vi "Test DMM Module API.vi"() -> ()   [LabVIEW 2018]
doc: "DMM Module API Tester."
uses:
  DMM Module.lvlib
  Application/Application.lvlib
panel:
  out "range?":string
  in  "query range":bool
  out "func?":string
  in  "Query func":bool
  in  "DMM reset":bool
  in  "DMM connect and reset":bool
  in  "Sets to Display":u16(ring)=2 items=["1st Display", "2nd Display", "1st & 2nd Display"]
  out "DCI":dbl
  out "DCV":dbl
  in  "DMM Close":bool
  in  "Detector Rate":u8(ring)=2 items=["SLOW", "MID", "FAST"]
  in  "DCI range":dbl=0.5 format="%#_13g"
  in  "DCV range":dbl=1000.0
  in  "Read DCV_DCI":bool
  in  "config channel":bool
  in  "DMM name":refnum<visa-resource-name>="COM15"
  in  "Show Block Diagram":bool
  in  "Stop Module":bool
  in  "Start Module":bool
  in  "Hide Module Panel":bool
  in  "Show Module Panel":bool
  out "Status":string
  out "Module Running?":bool
  # "This VI tests the API for the Module."
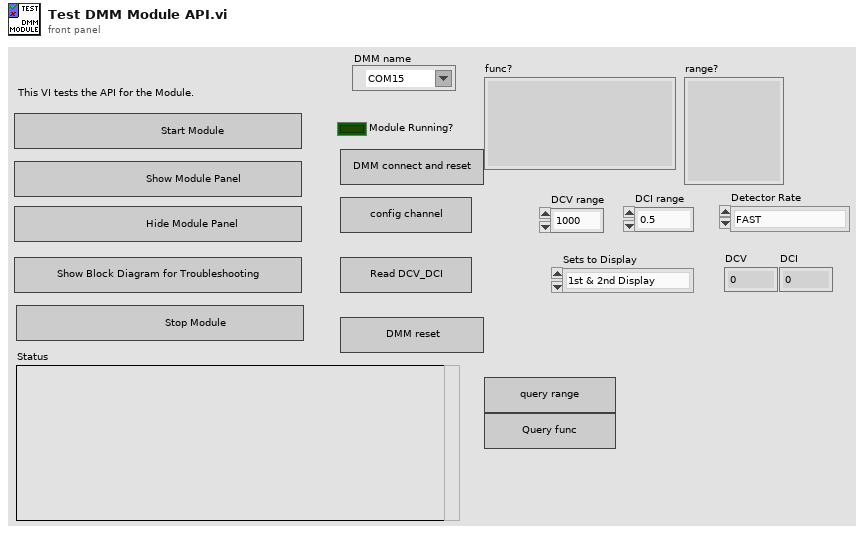
[diagram p1: front panel]
types:
  T1 = typedef "DMM Module.lvlib/Broadcast Events--cluster.ctl" = cluster{"Module Did Init":refnum<user-event>, "Status Updated":refnum<user-event>, "Error Reported":refnum<user-event>, "Module Did Stop":refnum<user-event>, "Update Module Execution Status":refnum<user-event>}
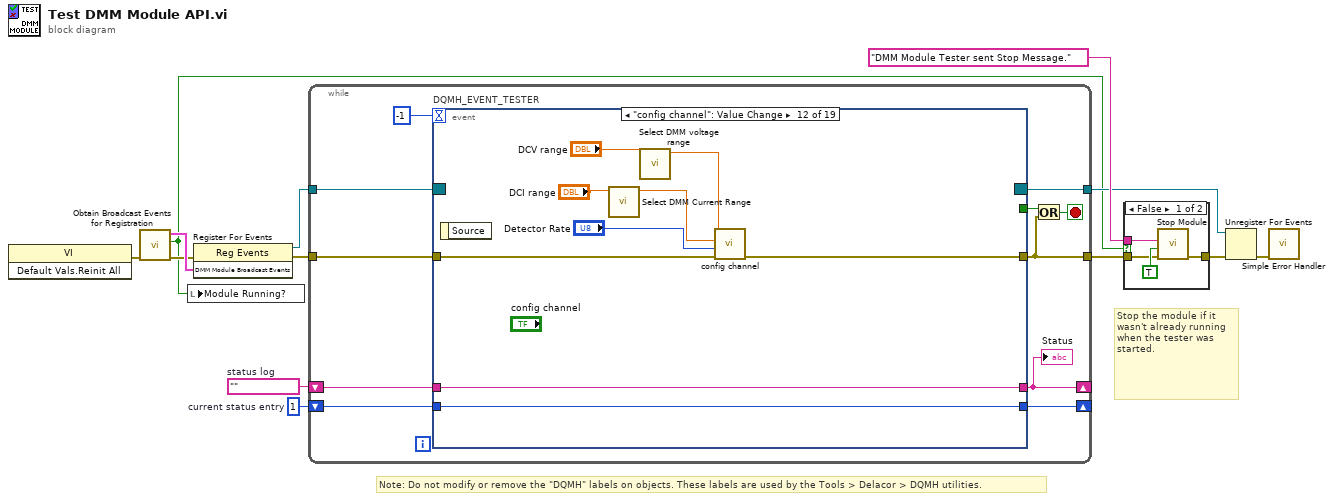
[diagram p0: block diagram]
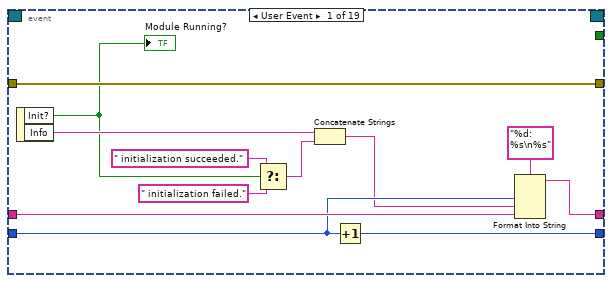
[diagram p3: hidden frame]
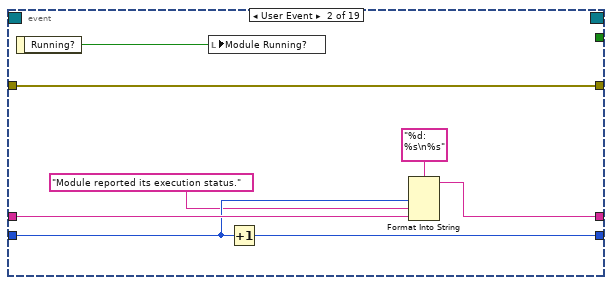
[diagram p4: hidden frame]
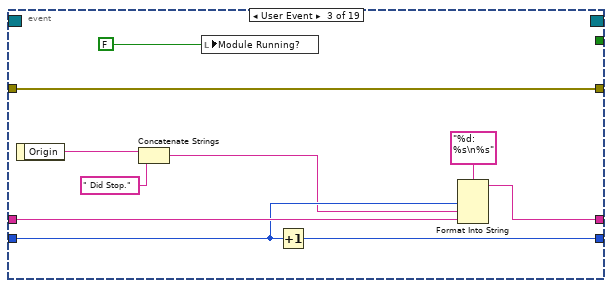
[diagram p5: hidden frame]
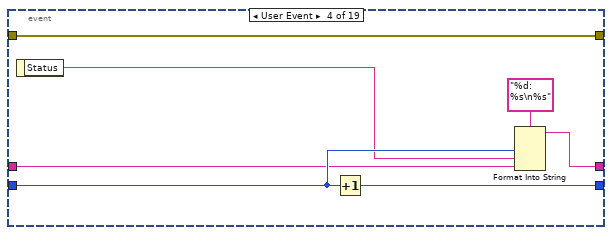
[diagram p6: hidden frame]
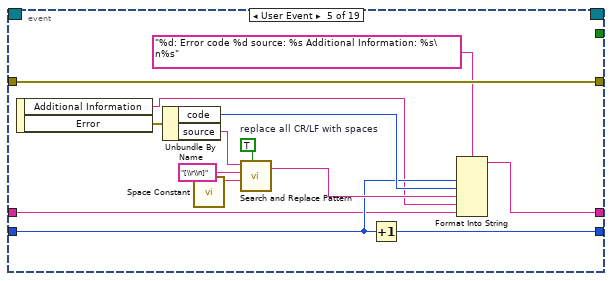
[diagram p7: hidden frame]
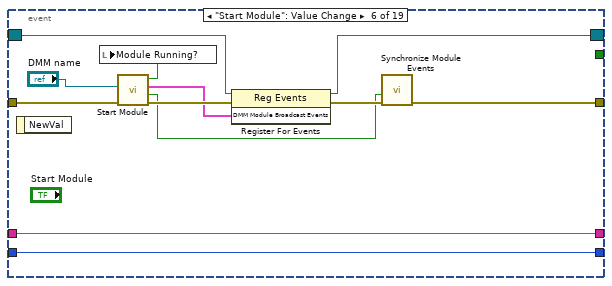
[diagram p8: hidden frame]
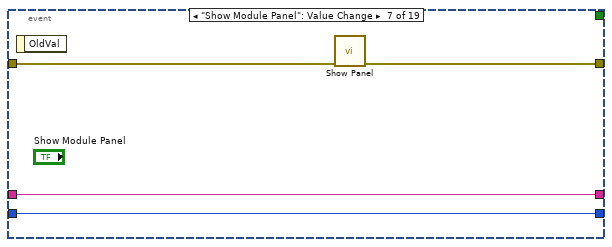
[diagram p9: hidden frame]
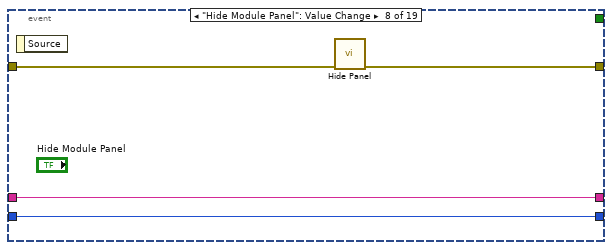
[diagram p10: hidden frame]
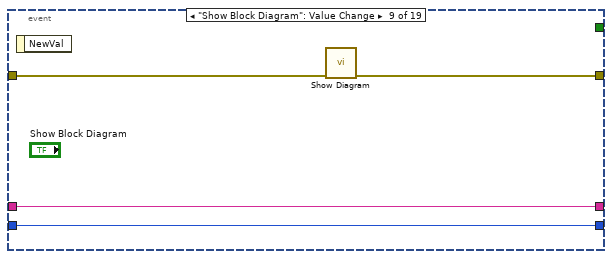
[diagram p11: hidden frame]
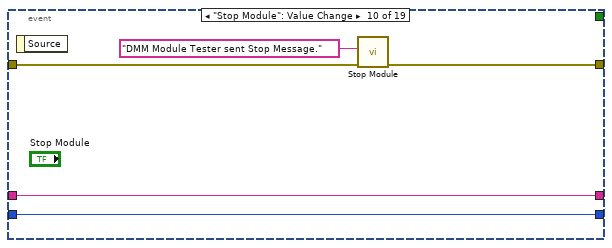
[diagram p12: hidden frame]
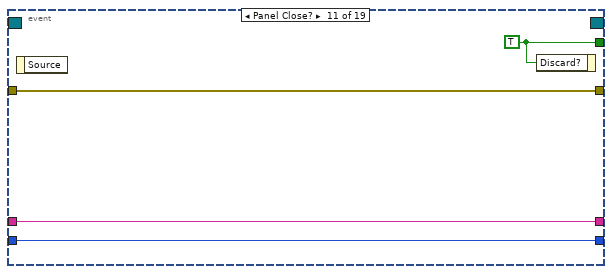
[diagram p13: hidden frame]
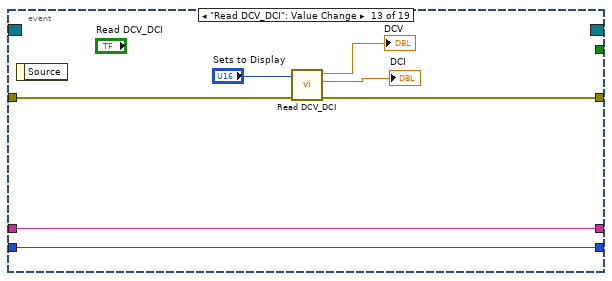
[diagram p14: hidden frame]
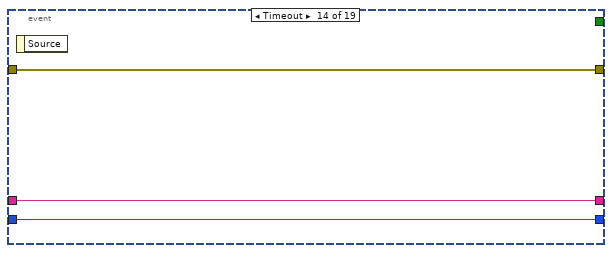
[diagram p15: hidden frame]
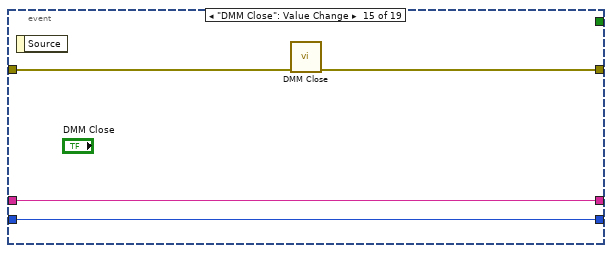
[diagram p16: hidden frame]
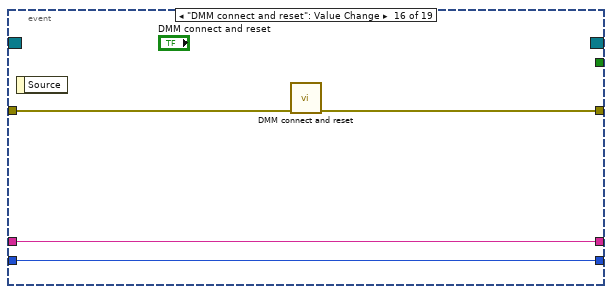
[diagram p17: hidden frame]
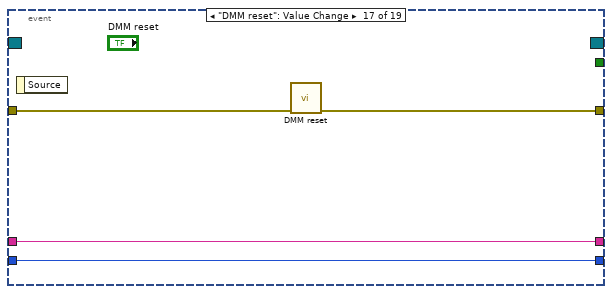
[diagram p18: hidden frame]
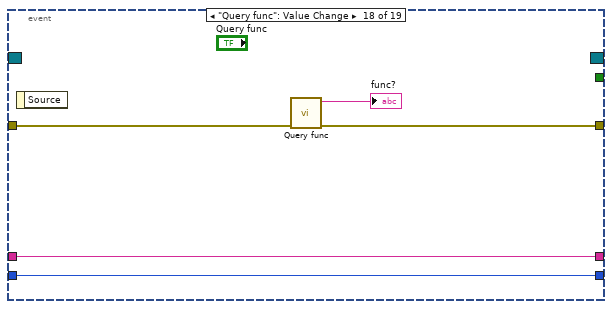
[diagram p19: hidden frame]
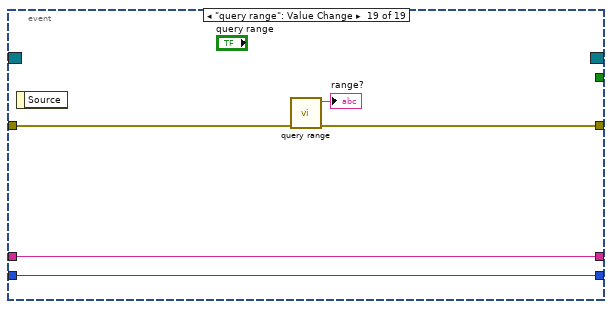
[diagram p20: hidden frame]
diagram:
  w10 = 1  # current status entry
  w11 = ""  # status log
  # "Stop the module if it wasn't already running when the tester was started."
  # "Note: Do not modify or remove the \"DQMH\" labels on objects. These labels are used by the Tools > Delacor > DQMH utilities."
  n1 = invoke class="VI" method="Default Vals.Reinit All"() -> (error out=w5:errorcluster)  [unwired: 3 in, 2 out]
  n2 = call "Obtain Broadcast Events for Registration.vi"("error in (no error)"=w5) -> ("error out"=w4:errorcluster, "Already running?"=w3:bool, "DMM Module Broadcast Events"=w8:T1)  [unwired: 8 in]
  n3 = local write "Module Running?"(w3) -> ()
  n4 = register-events(error in=w4, w8) -> (reference out=w7:refnum<event-registration>, error out=w9:errorcluster)  [unwired: 1 in]
  n5 = while {
    tunnel: w7 -> [w24]
    tunnel: [w15] -> w2
    shift-right: [w19] -> _
    shift-left: w11 -> [w21]
    shift-right: [w20] -> _
    shift-left: w10 -> [w22]
    tunnel: w9 -> [w17]
    tunnel: [w16] -> w6
    stop <- w18 stop-if-true
    n6 = event "DQMH_EVENT_TESTER" shown="[11] \"config channel\": Value Change" {
      selector: w24 -> [_ _ _ _ _ w81 _ _ _ _ _ _ _ _ _ _ _ _ _]
      dyn-events: [_ _ _ _ _ w80 _ _ _ _ _ _ _ _ _ _ _ _ _] -> w16
      timeout: -1 -> [_ _ _ _ _ _ _ _ _ _ _ _ _ _ _ _ _ _ _]
      tunnel: [_ _ _ _ _ _ _ _ _ _ w108 _ _ _ _ _ _ _ _] -> w23
      tunnel: [w36 w38 w45 w55 w75 w79 w91 w95 w96 w102 w105 w114 w118 w125 w128 w132 w136 w141 w146] -> w15
      tunnel: w22 -> [w33 w42 w52 w58 w65 w84 w89 w93 w97 w103 w106 w115 w123 w126 w129 w133 w137 w142 w147]
      tunnel: w21 -> [w34 w43 w53 w57 w63 w85 w90 w94 w98 w104 w107 w116 w124 w127 w130 w134 w138 w143 w148]
      tunnel: [w31 w40 w50 w59 w66 w85 w90 w94 w98 w104 w107 w116 w124 w127 w130 w134 w138 w143 w148] -> w19
      tunnel: [w32 w41 w51 w61 w64 w84 w89 w93 w97 w103 w106 w115 w123 w126 w129 w133 w137 w142 w147] -> w20
      tunnel: w17 -> [w36 w38 w45 w55 w75 w78 w88 w92 w99 w100 w105 w117 w119 w125 w131 w135 w139 w144 w149]
      event User Event {
        n7 = event-data() -> ("Init?"=w28:bool, "Info"=w30:string)  [unwired: 1 in]
        "Module Running?" <- w28
        n8 = Select(t=" initialization succeeded.", s=w28, f=" initialization failed.") -> (s? t:f=w25:string)
        n9 = Concatenate Strings(w30, w25) -> (w29:string)
        n10 = Increment(x=w33) -> (x+1=w32:i32)
        n11 = Format Into String(format string="%d: %s\n%s", w33, w29, w34) -> (resulting string=w31:string)  [unwired: 2 in, 1 out]
      }
      event User Event {
        n12 = event-data() -> ("Running?"=w37:bool)  [unwired: 1 in]
        n13 = local write "Module Running?"(w37) -> ()
        n14 = Increment(x=w42) -> (x+1=w41:i32)
        n15 = Format Into String(format string="%d: %s\n%s", w42, "Module reported its execution status.", w43) -> (resulting string=w40:string)  [unwired: 2 in, 1 out]
      }
      event User Event {
        n16 = event-data() -> ("Origin"=w49:string)  [unwired: 1 in]
        n17 = Concatenate Strings(w49, " Did Stop.") -> (w48:string)
        n18 = local write "Module Running?"(FALSE ("Module Did Init?")) -> ()
        n19 = Increment(x=w52) -> (x+1=w51:i32)
        n20 = Format Into String(format string="%d: %s\n%s", w52, w48, w53) -> (resulting string=w50:string)  [unwired: 2 in, 1 out]
      }
      event User Event {
        n21 = event-data() -> ("Status"=w56:string)  [unwired: 1 in]
        n22 = Increment(x=w58) -> (x+1=w61:i32)
        n23 = Format Into String(format string="%d: %s\n%s", w58, w56, w57) -> (resulting string=w59:string)  [unwired: 2 in, 1 out]
      }
      event User Event {
        w71 = TRUE  # replace all CR/LF with spaces
        n24 = event-data() -> ("Additional Information"=w62:string, "Error"=w67:errorcluster)  [unwired: 1 in]
        n25 = Unbundle By Name(w67) -> ("code"=w68:i32, "source"=w69:string)
        n26 = call <vilib>:"Space Constant.vi"() -> ("String"=w72:string)
        n27 = call <vilib>:"Search and Replace Pattern.vi"("string"=w69, "regular expression (\"\")"="[\\r\\n]" ("regular expression (\"\")"), "replace string (\"\")"=w72, "replace all? (F)"=w71) -> ("result string"=w70:string)  [unwired: 1 in, 1 out]
        n28 = Increment(x=w65) -> (x+1=w64:i32)
        n29 = Format Into String(format string="%d: Error code %d source: %s Additional Information: %s\n%s", w65, w68, w70, w62, w63) -> (resulting string=w66:string)  [unwired: 2 in, 1 out]
      }
      event "Start Module": Value Change {
        n30 = event-data() -> ()  [unwired: 1 in, 1 out]
        n31 = call "Start Module.vi"("error in (no error)"=w78, "VISA resource name 2"="DMM name") -> ("error out"=w86:errorcluster, "Wait for Event Sync?"=w83:bool, "DMM Module Broadcast Events"=w82:T1, "Module Was Already Running?"=w77:bool)  [unwired: 6 in]
        n32 = local write "Module Running?"(w77) -> ()
        n33 = register-events(reference=w81, error in=w86, w82) -> (reference out=w80:refnum<event-registration>, error out=w87:errorcluster)
        n34 = call "Synchronize Module Events.vi"("error in"=w87, "Wait for Event Sync?"=w83) -> ("error out"=w79:errorcluster)  [unwired: 9 in]
      }
      event "Show Module Panel": Value Change {
        n35 = event-data() -> ()  [unwired: 1 in, 1 out]
        n36 = call "Show Panel.vi"("error in (no error)"=w88) -> ("error out"=w91:errorcluster)  [unwired: 10 in]
      }
      event "Hide Module Panel": Value Change {
        n37 = event-data() -> ()  [unwired: 1 in, 1 out]
        n38 = call "Hide Panel.vi"("error in (no error)"=w92) -> ("error out"=w95:errorcluster)  [unwired: 10 in]
      }
      event "Show Block Diagram": Value Change {
        n39 = event-data() -> ()  [unwired: 1 in, 1 out]
        n40 = call "Show Diagram.vi"("error in (no error)"=w99) -> ("error out"=w96:errorcluster)  [unwired: 10 in]
      }
      event "Stop Module": Value Change {
        n41 = event-data() -> ()  [unwired: 1 in, 1 out]
        n42 = call "Stop Module.vi"("error in"=w100, "Origin"="DMM Module Tester sent Stop Message.") -> ("error out"=w102:errorcluster)  [unwired: 9 in]
      }
      event Panel Close? {
        w108 = TRUE ("Discard?")
        n43 = event-data() -> ()  [unwired: 1 in, 1 out]
        n44 = event-data("Discard?"=w108) -> ()  [unwired: 1 in, 1 out]
      }
      event "config channel": Value Change {
        n45 = event-data() -> ()  [unwired: 1 in, 1 out]
        n46 = call "Select DMM Current Range.vi"("Max"="DCI range") -> ("DMM current range"=w111:dbl)  [unwired: 8 in, 2 out]
        n47 = call "Select DMM voltage range.vi"("Max"="DCV range") -> ("DDM voltage Range"=w109:dbl)  [unwired: 9 in, 1 out]
        n48 = call "config channel.vi"("error in"=w117, "Detector Rate"="Detector Rate", "DCI range"=w111, "DCV range"=w109) -> ("error out"=w114:errorcluster)  [unwired: 7 in]
      }
      event "Read DCV_DCI": Value Change {
        n49 = event-data() -> ()  [unwired: 1 in, 1 out]
        n50 = call "Read DCV_DCI.vi"("error in"=w119, "Sets to Display"="Sets to Display") -> ("error out"=w118:errorcluster, "DCI"=→"DCI":dbl, "DCV"=→"DCV":dbl)  [unwired: 6 in, 1 out]
      }
      event Timeout {
        n51 = event-data() -> ()  [unwired: 1 in, 1 out]
      }
      event "DMM Close": Value Change {
        n52 = event-data() -> ()  [unwired: 1 in, 1 out]
        n53 = call "DMM Close.vi"("error in"=w131) -> ("error out"=w128:errorcluster)  [unwired: 10 in]
      }
      event "DMM connect and reset": Value Change {
        n54 = event-data() -> ()  [unwired: 1 in, 1 out]
        n55 = call "DMM connect and reset.vi"("error in"=w135) -> ("error out"=w132:errorcluster)  [unwired: 10 in]
      }
      event "DMM reset": Value Change {
        n56 = event-data() -> ()  [unwired: 1 in, 1 out]
        n57 = call "DMM reset.vi"("error in"=w139) -> ("error out"=w136:errorcluster)  [unwired: 10 in]
      }
      event "Query func": Value Change {
        n58 = event-data() -> ()  [unwired: 1 in, 1 out]
        n59 = call "Query func.vi"("error in"=w144) -> ("error out"=w141:errorcluster, "String"=→"func?":string)  [unwired: 8 in, 1 out]
      }
      event "query range": Value Change {
        n60 = event-data() -> ()  [unwired: 1 in, 1 out]
        n61 = call "query range.vi"("error in"=w149) -> ("error out"=w146:errorcluster, "String"=→"range?":string)  [unwired: 8 in, 1 out]
      }
    }
    "Status" <- w19
    n62 = Or(x=w23, y=w15) -> (x .or. y?=w18:bool)
  }
  n63 = case shown="False" w3 {
    tunnel: [w153 w154] -> w13
    tunnel: "DMM Module Tester sent Stop Message." ("Origin") -> [w152 _]
    tunnel: w2 -> [w150 w154]
    frame False {
      n64 = call "Stop Module.vi"("error in"=w150, "Wait for Module to Stop? (F)"=TRUE ("Wait for Module to stop?"), "Origin"=w152) -> ("error out"=w153:errorcluster)  [unwired: 8 in]
    }
    frame True {
    }
  }
  n65 = Unregister For Events(event registration refnum=w6, error in=w13) -> (error out=w1:errorcluster)
  n66 = call <vilib>:"Simple Error Handler.vi"("error in (no error)"=w1) -> ()  [unwired: 4 in, 5 out]
